vi "DAQmx Start Trigger (Digital Edge).vi"(0 "task/channels in":refnum<k21>, 5 "source":tag, 7 "edge":i32(ring)=10280 items=["Rising"=10280, "Falling"=10171], 11 "error in":errorcluster) -> (4 "task out":refnum<k21>, 15 "error out":errorcluster)   [LabVIEW 2011]
doc: "Configures the task to start acquiring or generating samples on a rising or falling edge of a digital signal."
uses:
  C:/Program Files/National Instruments/LabVIEW 2011/resource/objmgr/daqmx.rc
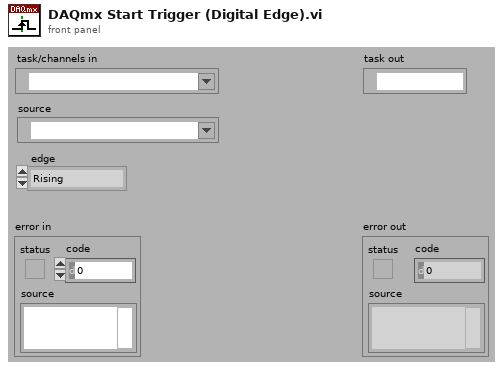
[diagram p1: front panel]
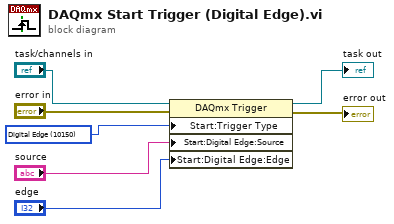
[diagram p0: block diagram]
diagram:
  w2 = 10150 items=["Analog Edge"=10099, "Digital Edge"=10150, "Analog Window"=10103, "None"=10230] ("Start:Trigger Type")
  n1 = property class="DAQmx Trigger"(reference="task/channels in", error in="error in", "Start:Trigger Type"=w2, "Start:Digital Edge:Source"="source", "Start:Digital Edge:Edge"="edge") -> (reference out=→"task out":refnum<k21>, error out=→"error out":errorcluster)
